vi "K2400_I_Protection.vi"(2 "error in":errorcluster, 3 "Comp (mA)":dbl format="%#_3g", 4 "address (24)":string) -> (0 "error out":errorcluster)   [LabVIEW 2021]
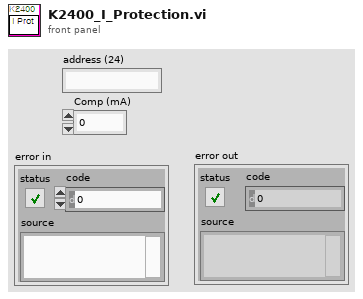
[diagram p1: front panel]
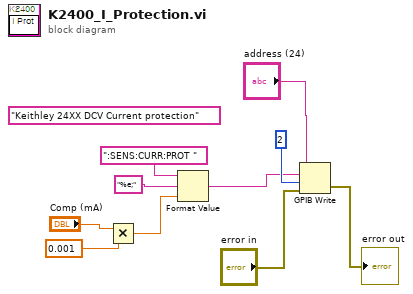
[diagram p0: block diagram]
diagram:
  (unwired) "Keithley 24XX DCV Current protection"
  n1 = Multiply(x="Comp (mA)", y=0.001) -> (x*y=w3:dbl)
  n2 = Format Value(string ("")=":SENS:CURR:PROT ", format string="%e;", value (0)=w3) -> (output string=w9:string)
  n3 = GPIB Write(0:"address (24)", 1:w9, 2:2, 3:"error in") -> (6:→"error out":errorcluster)  [unwired: 1 in, 1 out]
